vi "Soft Serial-Read RAW GPS UART.vi"   [LabVIEW 2014]
uses:
  PWS_ESP8266/PWS_ESP8266.lvlib
panel:
  # "Overview: Demonstrates how to read GPS data from Pmod GPS, This example using Soft Serial API to communicate with UART PmodGPS, Because PWS's onboard serial port will be using for debuging the data from PmodGPS.\nRequirements: LabVIEW Full Development System,Arduino Compatible Compiler for LabVIEW,Programmable Wireless Stamp (PWS) Library.\nInstructions:\n1. Plug-in PmodGPS  to SPI port refer diagram below. (It is NOT using SPI bus, But this example will using GPIO as a Soft Serial pins)\n2.  If this example has been loaded from the Arduino Compatible Compiler for LabVIEW, simply select Compile and Download.  Otherwise, open Tools>Arduino Compatible Compiler for LabVIEW in LabVIEW, then select File>Load VI, and select this VI and then Compile and Download.\n3. Open \"Serial Monitor\" by select \"Tools>Serial Monitor\" and select baud rate to 9600.\n4. Observe the logged data being print out on serial port monitor. \n\n#NOTE: \nThe PmodGPS is an ideal solution for any embedded system in need of satellite positioning accuracy. It features the GlobalTop Gms-u1LP GPS antenna module which utilizes the MediaTek GPS MT3329. refer : https://digilentinc.com/Products/Detail.cfm?Prod=PMOD-GPS"
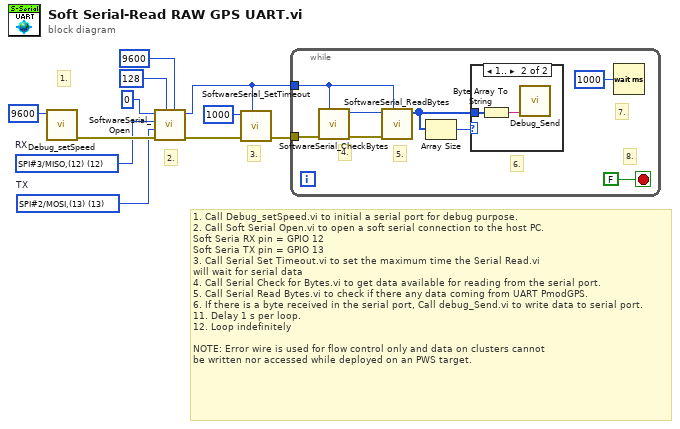
[diagram p0: block diagram]
diagram:
  w1 = u8 13 items=["SPI#1/SS,(5)"=5, "SPI#2/MOSI,(13)"=13, "SPI#3/MISO,(12)"=12, "SPI#4/SCLK,(14)"=14, "UART#1/CS,(15)"=15, "UART#2/TXD,(1)"=1, "UART#3/RXD,(3)"=3, "UART#4/LED,(16)"=16, "FPROM_Btn,(0)"=0, "SDCard_CS,(4)"=4, "I2C-SDA/TXD1,(2)"=2, "ADC0,(17)"=17]  # TX
  w2 = u8 12 items=["SPI#1/SS,(5)"=5, "SPI#2/MOSI,(13)"=13, "SPI#3/MISO,(12)"=12, "SPI#4/SCLK,(14)"=14, "UART#1/CS,(15)"=15, "UART#2/TXD,(1)"=1, "UART#3/RXD,(3)"=3, "UART#4/LED,(16)"=16, "FPROM_Btn,(0)"=0, "SDCard_CS,(4)"=4, "I2C-SDA/TXD1,(2)"=2, "ADC0,(17)"=17]  # RX
  # "1. Call Debug_setSpeed.vi to initial a serial port for debug purpose.\n2. Call Soft Serial Open.vi to open a soft serial connection to the host PC.\nSoft Seria RX pin = GPIO 12\nSoft Seria TX pin = GPIO 13\n3. Call Serial Set Timeout.vi to set the maximum time the Serial Read.vi\nwill wait for serial data\n4. Call Serial Check for Bytes.vi to get data available for reading from the serial port. \n5. Call Serial Read Bytes.vi to check if there any data coming from UART PmodGPS.\n6. If there is a byte received in the serial port, Call debug_Send.vi to write data to serial port.\n11. Delay 1 s per loop.\n12. Loop indefinitely\n\nNOTE: Error wire is used for flow control only and data on clusters cannot\nbe written nor accessed while deployed on an PWS target."
  # "3."
  # "2."
  # "1."
  n1 = call "Debug_setSpeed.vi"("Speed"=u32 9600) -> ("error out"=w8:errorcluster)  [unwired: 10 in]
  n2 = call "SoftwareSerial_Open.vi"("Speed"=u32 9600, "Buffer"=u8 128, "error in (no error)"=w8, "Tx"=w1, "Rx"=w2, "Interface (0-4)"=u8 0) -> ("error out"=w6:errorcluster, "Instance"=w4:u8)  [unwired: 4 in]
  n3 = call "SoftwareSerial_SetTimeout.vi"("Instance"=w4, "error in (no error)"=w6, "Timeout (ms)"=1000) -> ("error out"=w5:errorcluster)  [unwired: 8 in]
  n4 = while {
    tunnel: w5 -> [w17]
    tunnel: w4 -> [w14]
    stop <- FALSE stop-if-true
    # "8."
    # "7."
    # "6."
    # "5."
    # "4."
    n5 = call "SoftwareSerial_CheckBytes.vi"("Instance"=w14, "error in (no error)"=w17) -> ("error out"=w16:errorcluster, "Bytes"=w15:i32)  [unwired: 8 in]
    n6 = call "SoftwareSerial_ReadBytes.vi"("Instance"=w14, "error in (no error)"=w16, "Length"=w15) -> ("Data"=w13:u8[])  [unwired: 6 in, 2 out]
    n7 = Array Size(array=w13) -> (size(s)=w12:i32)
    n8 = case shown="1.." w12 {
      tunnel: w13 -> [_ w21]
      frame 0, Default {
      }
      frame 1.. {
        n9 = Byte Array To String(unsigned byte array=w21) -> (string=w20:string)
        n10 = call "Debug_Send.vi"("DATA"=w20) -> ()  [unwired: 11 in]
      }
    }
    n11 = Wait (ms)(milliseconds to wait=u32 1000) -> ()  [unwired: 1 out]
  }
